vi "S2C_5190CR_Proc_TcpRead.vi"(7 "Line Seperator":string="\\n", 8 "Error In":errorcluster, 9 "Timeout(ms)":i32, 10 "Bytes":i32, 11 "Read Mode":enum16{"Normal", "Line"}(ring)) -> (0 "Error Out":errorcluster, 3 "Data":string)   [LabVIEW 2015]
doc: "Performs a TCP read."
uses:
  S2C_5190CR_Proc_Globals.vi
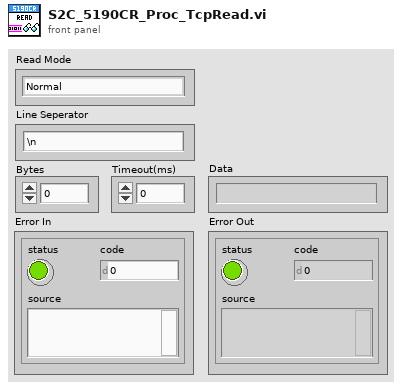
[diagram p1: front panel]
types:
  T1 = enum16{"Standard", "Buffered", "CRLF", "Immediate"}
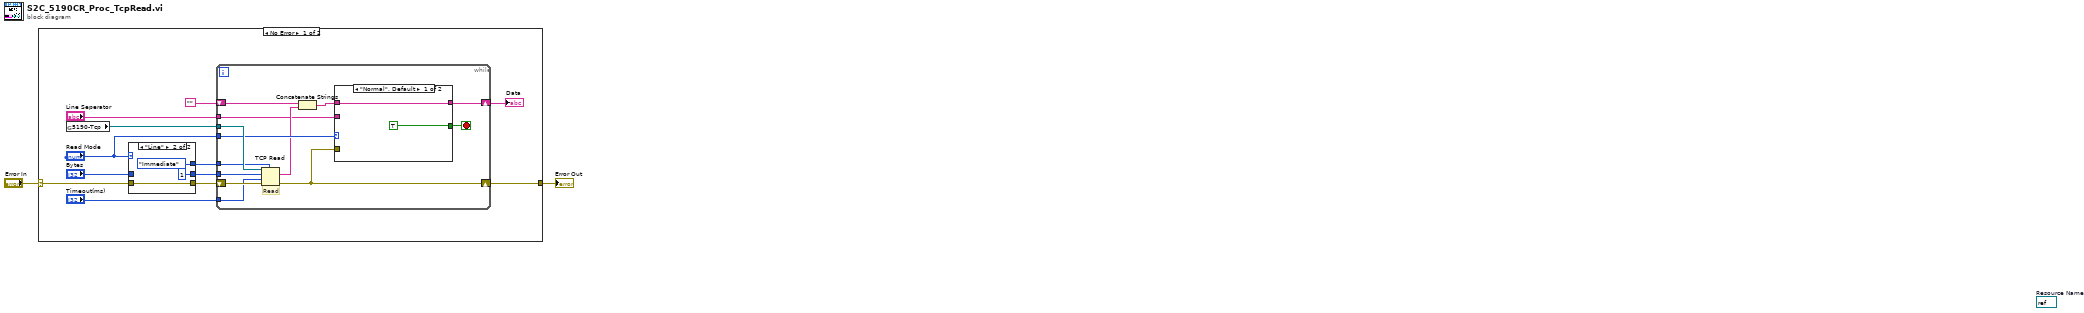
[diagram p0: block diagram]
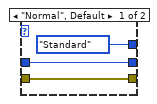
[diagram p2: hidden frame]
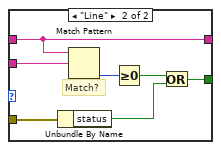
[diagram p3: hidden frame]
diagram:
  (unwired) refnum<visa-resource-name> refnum  # Resource Name
  n1 = case shown="No Error" "Error In" {
    selector: "Error In" -> [w8 w43]
    tunnel: [w4 w43] -> w1
    frame No Error {
      n2 = global read "S2C_5190CR_Proc_Globals.vi" "5190-Tcp"() -> (w12:refnum<k5>)
      n3 = case shown="\"Line\"" "Read Mode" {
        tunnel: "Bytes" -> [w17 _]
        tunnel: [w17 1 ("Bytes")] -> w11
        tunnel: [T1."Standard" ("mode (standard)") T1."Immediate" ("mode (standard)")] -> w10
        tunnel: w8 -> [w15 w18]
        tunnel: [w15 w18] -> w7
        frame "Normal", Default {
        }
        frame "Line" {
        }
      }
      n4 = while {
        tunnel: "Timeout(ms)" -> [w32]
        tunnel: w12 -> [w31]
        tunnel: w11 -> [w30]
        tunnel: w10 -> [w29]
        tunnel: "Read Mode" -> [w28]
        shift-right: [w24] -> w3
        shift-left: "" -> [w27]
        shift-right: [w22] -> w4
        shift-left: w7 -> [w33]
        tunnel: "Line Seperator" -> [w23]
        stop <- w21 stop-if-true
        # "Read"
        n5 = TCP Read(connection ID=w31, bytes to read=w30, error in (no error)=w33, 7:w29, 9:w32) -> (data out=w26:string, error out=w22:errorcluster)  [unwired: 1 out]
        n6 = Concatenate Strings(w27, w26) -> (w25:string)
        n7 = case shown="\"Normal\", Default" w28 {
          tunnel: w25 -> [w35 w42]
          tunnel: [w35 w42] -> w24
          tunnel: w23 -> [_ w41]
          tunnel: w22 -> [_ w39]
          tunnel: [TRUE w36] -> w21
          frame "Normal", Default {
          }
          frame "Line" {
            # "Match?"
            n8 = Unbundle By Name(w39) -> ("status"=w37:bool)
            n9 = Match Pattern(string=w42, regular expression=w41) -> (offset past match=w40:i32)  [unwired: 1 in, 3 out]
            n10 = Greater Or Equal To 0?(x=w40) -> (x >= 0?=w38:bool)
            n11 = Or(x=w38, y=w37) -> (x .or. y?=w36:bool)
          }
        }
      }
      "Data" <- w3
    }
    frame Error {
    }
  }
  "Error Out" <- w1
